vi "24位RGB灰度图(何-老设备)转换为8位灰度图子VI.vi"(11 "File Path":path) -> (0 "原始图像":T1, 2 "转换后的原始图像":T1(plugin-control), 3 "Path":path)   [LabVIEW 2018]
uses:
  <vilib>/vision/Image Controls.llb/IMAQ Image.ctl
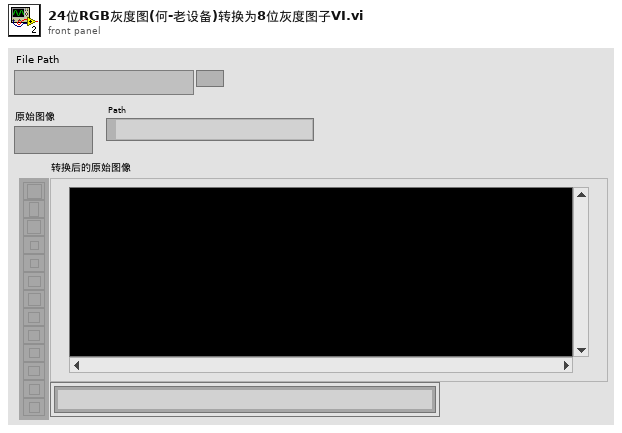
[diagram p1: front panel]
types:
  T1 = typedef "IMAQ Image.ctl" = refnum<image>
  T2 = typedef "Image Type" = u32
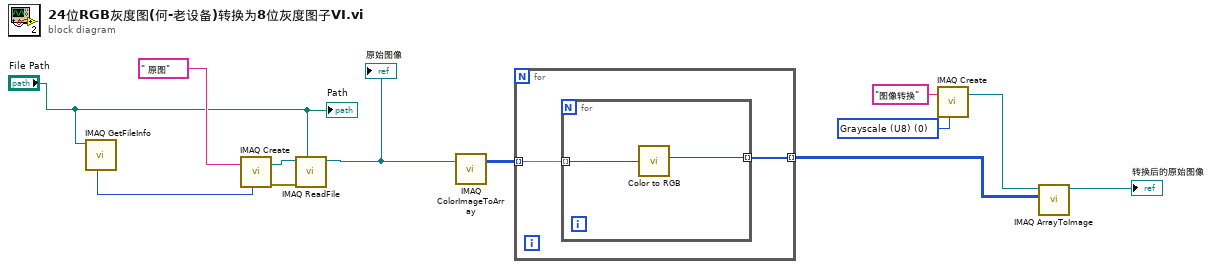
[diagram p0: block diagram]
diagram:
  w10 = T2 0 items=["Grayscale (U8)", "Grayscale (I16)", "Grayscale (SGL)", "Complex (CSG)", "RGB (U32)", "HSL (U32)", "RGB (U64)", "Grayscale (U16)"] ("Image Type")
  n1 = call "IMAQ GetFileInfo"("File Path"="File Path") -> ("Image Type"=w3:T2)  [unwired: 4 in, 6 out]
  n2 = call "IMAQ Create"("Image Name"=" 原图", "Image Type"=w3) -> ("New Image"=w4:T1, "error out"=w5:errorcluster)  [unwired: 3 in]
  n3 = call "IMAQ ReadFile"("File Path"="File Path", "error in (no error)"=w5, "Image"=w4) -> ("Image Out"=w2:T1)  [unwired: 4 in, 4 out]
  "原始图像" <- w2
  n4 = call "IMAQ ColorImageToArray"("Image"=w2) -> ("Image Pixels (U32)"=w12:u32[][])  [unwired: 3 in, 2 out]
  n5 = for {
    tunnel: w12 -> [w14] mode=indexing
    tunnel: [w13] -> w8 mode=indexing
    n6 = for {
      tunnel: w14 -> [w16] mode=indexing
      tunnel: [w15] -> w13 mode=indexing
      n7 = call <vilib>:"Color to RGB.vi"("Color"=w16) -> ("R"=w15:u8)  [unwired: 3 out]
    }
  }
  n8 = call "IMAQ Create"("Image Name"="图像转换", "Image Type"=w10) -> ("New Image"=w9:T1)  [unwired: 3 in, 1 out]
  n9 = call "IMAQ ArrayToImage"("Image Pixels (U8)"=w8, "Image"=w9) -> ("Image Out"=→"转换后的原始图像":T1)  [unwired: 8 in, 1 out]
  "Path" <- "File Path"
